vi "isMoving.vi"(3 "Device in":refnum<k24>) -> (1 "IsMoving":bool)   [LabVIEW 2014]
doc: "André Romero - 2017\nandretec@ifsc.usp.br"
uses:
  C:/UserLabs/Andre/kinesis-lab14-32bits/kinesis-teste/Kinesis/Thorlabs.MotionControl.TCube.DCServoCLI.dll
  Kinesis/Thorlabs.MotionControl.TCube.DCServoCLI.dll
  C:/UserLabs/Andre/kinesis-lab14-32bits/kinesis-teste/Kinesis/Thorlabs.MotionControl.GenericMotorCLI.dll
  Kinesis/Thorlabs.MotionControl.GenericMotorCLI.dll
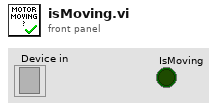
[diagram p1: front panel]
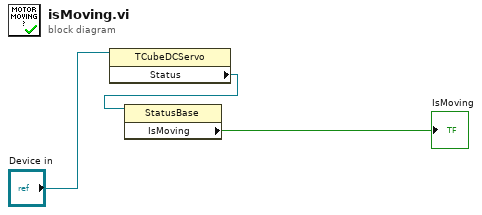
[diagram p0: block diagram]
diagram:
  n1 = property class="TCubeDCServo"(reference="Device in") -> ("Status"=w2:refnum<k24>)  [unwired: 1 in, 2 out]
  n2 = property class="StatusBase"(reference=w2) -> ("IsMoving"=→"IsMoving":bool)  [unwired: 1 in, 2 out]
